vi "Follow Path.vi"(0 "Drivetrain":T10, 1 "Encoder L":T6, 2 "Encoder R":T6, 3 "Gyro":T3 {"Sample Rate" min=0.25 max=100.0 step=0.25}, 4 "Trajectory":T1, 5 "error in":errorcluster, 6 "Queue in":refnum<queue>) -> (19 "error out":errorcluster)   [LabVIEW 2016, in "Drive System.lvlib"]
uses:
  Drive System.lvlib
  DriveCmd.ctl
  DriveCmdList.ctl
  <vilib>/Rock Robotics/WPI/RobotDrive/WPI_RobotDriveDevRef.ctl
  <vilib>/Rock Robotics/WPI/MotorControl/WPI_MotorControlDeviceRef.ctl
  <vilib>/Rock Robotics/WPI/MotorControl/WPI_MotorControlType.ctl
  <vilib>/Rock Robotics/SystemInterfaces/DIO/FPGA_DIOPWMChannel.ctl
  <vilib>/Rock Robotics/WPI/PWM/WPI_PWMDeadband.ctl
  <vilib>/Rock Robotics/WPI/Encoder/WPI_EncoderDevRef.ctl
  <vilib>/Rock Robotics/SystemInterfaces/Encoder/FPGA_EncoderIdx.ctl
  <vilib>/Rock Robotics/SystemInterfaces/Counter/FPGA_CounterCtrSystemIndex.ctl
  <vilib>/Rock Robotics/WPI/Encoder/WPI_EncoderType.ctl
  <vilib>/Rock Robotics/WPI/Gyro/WPI_GyroDevRef.ctl
  <vilib>/Rock Robotics/SystemInterfaces/AI/FPGA_AIChannel.ctl
  <vilib>/Rock Robotics/SystemInterfaces/spilib/spi_bus.ctl
  Varient Cmd Types/Follow Path.ctl
  Pathfinder/VIs/Segment.ctl
  <vilib>/Platform/TimedLoop/XDataNode/timing_clust.ctl
  <vilib>/Platform/TimedLoop/XDataNode/nitl_modes.ctl
  <vilib>/Platform/TimedLoop/XDataNode/wakeup.ctl
  Raw Data.vi
  <vilib>/Platform/TimedLoop/XDataNode/XDataNode.xnode
  <vilib>/Platform/TimedLoop/XDataNode/XDNodeRunTimeDep.lvlib
  Pathfinder/Pathfinder.lvlib
panel:
  in  "Gyro PIDF":cluster{"Kp":dbl, "Ki":dbl, "Kd":dbl, "Kf":dbl} {"Kf" format="%.3f"; "Kd" format="%.3f"; "Ki" format="%.3f"; "Kp" format="%.3f"}
  in  "Gyro iZone":dbl=inf format="%#_13g"
  in  "Gyro Invert":bool
  in  "Gyro output range":cluster{"output high":dbl, "output low":dbl}={"output high"=1.0, "output low"=-1.0} {"output low" format="%.2f"; "output high" format="%.2f"}
  in  "PIDF gains":cluster{"Kp":dbl, "Ki":dbl, "Kd":dbl, "Kf":dbl} {"Kf" format="%.3f"; "Kd" format="%.3f"; "Ki" format="%.3f"; "Kp" format="%.3f"}
  in  "i Zone":dbl=inf format="%.2f"
  in  "invert? (F)":bool
  in  "output range":cluster{"output high":dbl, "output low":dbl}={"output high"=1.0, "output low"=-1.0} {"output low" format="%.2f"; "output high" format="%.2f"}
  in  "Ka":dbl
  in  "Kv":dbl
  # "Analog"
  # "XRS"
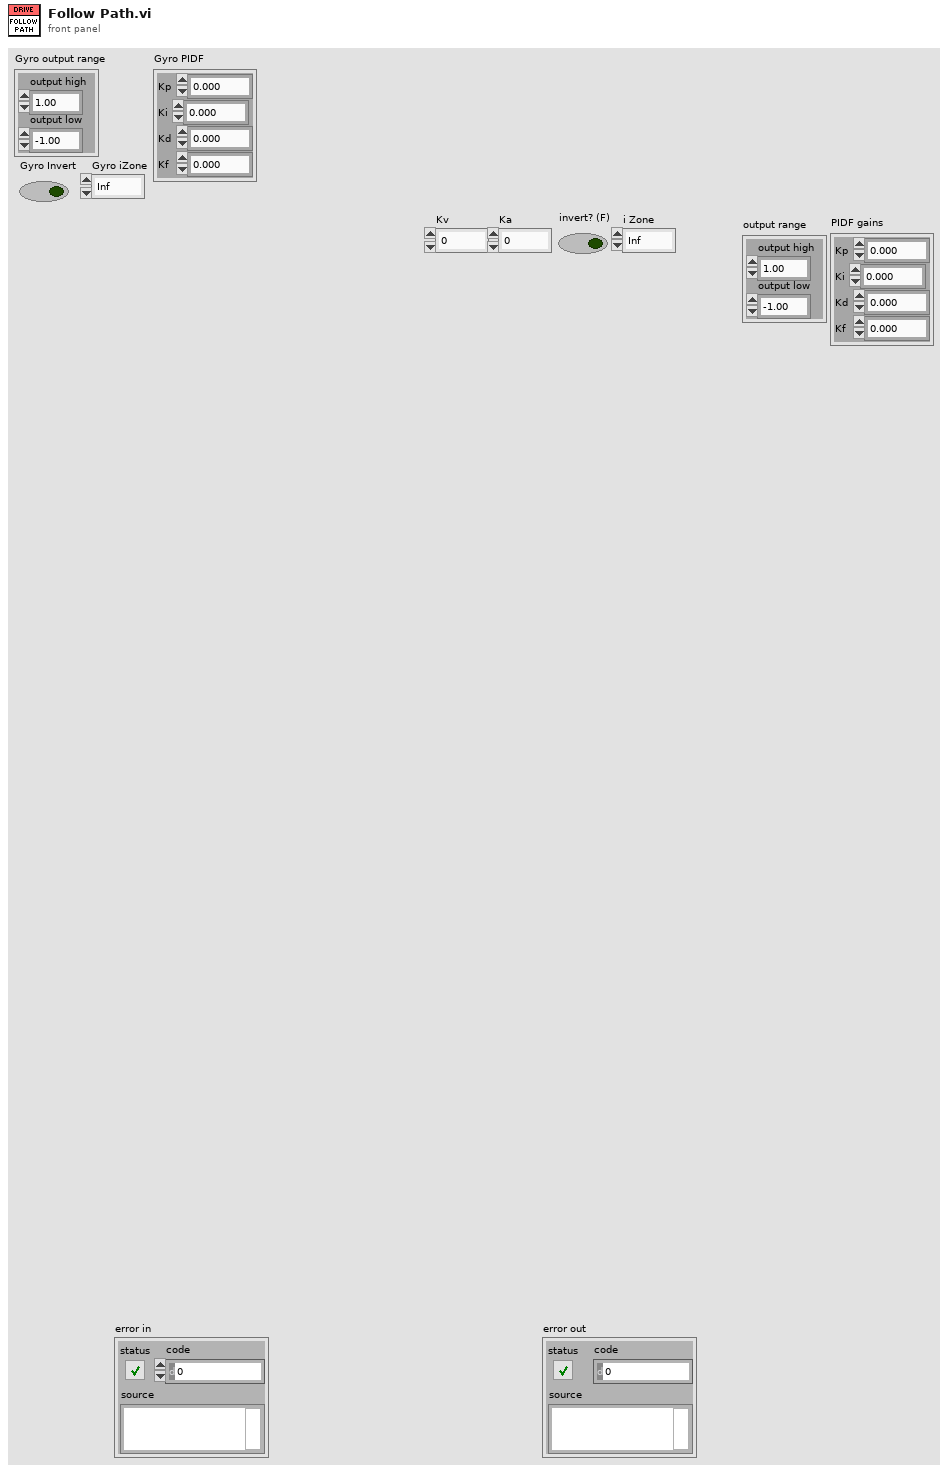
[diagram p1: front panel]
types:
  T1 = typedef "Drive System.lvlib/Follow Path.ctl" = cluster{"Left":T2[], "Right":T2[]}
  T2 = typedef "Pathfinder.lvlib/Segment.ctl" = cluster{"dt":dbl, "x":dbl, "y":dbl, "position":dbl, "velocity":dbl, "acceleration":dbl, "jerk":dbl, "heading":dbl}
  T3 = typedef "WPI_GyroDevRef.ctl" = cluster{"DevStatus":errorcluster, "Analog Channel":T4, "Offset":dbl, "Gain (VoltsPerDegree/Second)":dbl, "Gyro Type":enum16{"Analog", "XRS450"}, "Handle":i32, "SPI Bus":T5, "Device Found":bool, "Sample Rate":dbl, "Calibrate On Open":bool}
  T4 = typedef "FPGA_AIChannel.ctl" = enum8{"AI 0", "AI 1", "AI 2", "AI 3", "AI MXP 0", "AI MXP 1", "AI MXP 2", "AI MXP 3", "Invalid"}
  T5 = typedef "spi_bus.ctl" = enum16{"SPI On-Board, CS0", "SPI On-Board, CS1", "SPI On-Board, CS2", "SPI On-Board, CS3", "SPI MXP", "Invalid"}
  T6 = typedef "WPI_EncoderDevRef.ctl" = cluster{"DevStatus":errorcluster, "EncoderIndex":T7, "CounterIndex":T8, "DistancePerCount":dbl, "Decoding Type":T9}
  T7 = typedef "FPGA_EncoderIdx.ctl" = enum8{"Enc 0", "Enc 1", "Enc 2", "Enc 3", "Enc 4", "Enc 5", "Enc 6", "Enc 7", "Invalid"}
  T8 = typedef "FPGA_CounterCtrSystemIndex.ctl" = enum8{"Ctr 0", "Ctr 1", "Ctr 2", "Ctr 3", "Ctr 4", "Ctr 5", "Ctr 6", "Ctr 7", "Invalid"}
  T9 = typedef "WPI_EncoderType.ctl" = enum16{"1x", "2x", "4x"}
  T10 = typedef "WPI_RobotDriveDevRef.ctl" = cluster{"DevStatus":errorcluster, "Motors[]":T11[], "Square Inputs":bool, "Max Output":dbl}
  T11 = typedef "WPI_MotorControlDeviceRef.ctl" = cluster{"DeviceStatus":errorcluster, "Type":T12, "PWM":cluster{"PWM Channel":T13, "DeadBand":T14}, "CAN":cluster{"Device Number":u8, "SetOutput VI Ref":variant, "GetOutput VI Ref":variant, "Enable VI Ref":variant, "Disable VI Ref":variant, "Data":variant}, "Invert":bool}
  T12 = typedef "WPI_MotorControlType.ctl" = enum16{"PWM", "CAN"}
  T13 = typedef "FPGA_DIOPWMChannel.ctl" = enum8{"PWM 0", "PWM 1", "PWM 2", "PWM 3", "PWM 4", "PWM 5", "PWM 6", "PWM 7", "PWM 8", "PWM 9", "PWM MXP 0", "PWM MXP 1", "PWM MXP 2", "PWM MXP 3", "PWM MXP 4", "PWM MXP 5", "PWM MXP 6", "PWM MXP 7", "PWM MXP 8", "PWM MXP 9", "Invalid"}
  T14 = typedef "WPI_PWMDeadband.ctl" = cluster{"Name":string, "maxPositivePwm":i32, "minPositivePwm":i32, "centerPwm":i32, "maxNegativePwm":i32, "minNegativePwm":i32, "angularRange":u16}
  T15 = cluster{"Queue in":refnum<queue>, "Drivetrain":T10, "Encoder L":T6, "Encoder R":T6, "Gyro":T3}
  T16 = typedef "XDNodeRunTimeDep.lvlib/timing_clust.ctl" = cluster{"Expected End [f-1]":u64, "Actual End [f-1]":u64, "Finished Late? [f-1]":bool, "Expected End [i-1]":u64, "Actual End [i-1]":u64, "Finished Late? [i-1]":bool, "Expected Start [i]":u64, "Actual Start [i]":u64, "Expected Start [f]":u64, "Actual Start [f]":u64, "Source Name":string, "Structure Name":string, "Period":i64, "Deadline":i64, "Offset":i64, "Start":i64, "Priority":i32, "Timeout":i32, "Mode":T17, "Wakeup Reason":T18, "Error":errorcluster, "Source Type":string, "Secondary Source Type":string, "Global End Time":u64, "Global Start Time":u64, "Frame Duration":u64, "Iteration Duration":u64, "Assigned CPU":i32, "I/O Scan Engine Mode":u32}
  T17 = typedef "XDNodeRunTimeDep.lvlib/nitl_modes.ctl" = enum32{"No Change", "Process missed periods, maintain original phase", "Discard missed periods, maintain original phase", "Process missed periods, ignore original phase", "Discard missed periods, ignore original phase"}
  T18 = typedef "XDNodeRunTimeDep.lvlib/wakeup.ctl" = enum32{"Normal", "Aborted", "Asynchronous wakeup", "Timing source error", "Timed loop error", "Timeout"}
  T19 = typedef "Drive System.lvlib/DriveCmd.ctl" = cluster{"cmd":T20, "data":variant, "Force? (F)":bool, "Lock":string}
  T20 = typedef "Drive System.lvlib/DriveCmdList.ctl" = enum16{"Idle", "Cleanup", "Drive For Time", "Follow Path Speed Control", "Follow Path", "Drive Tank", "Drive Arcade", "Unlock", "Lock"}
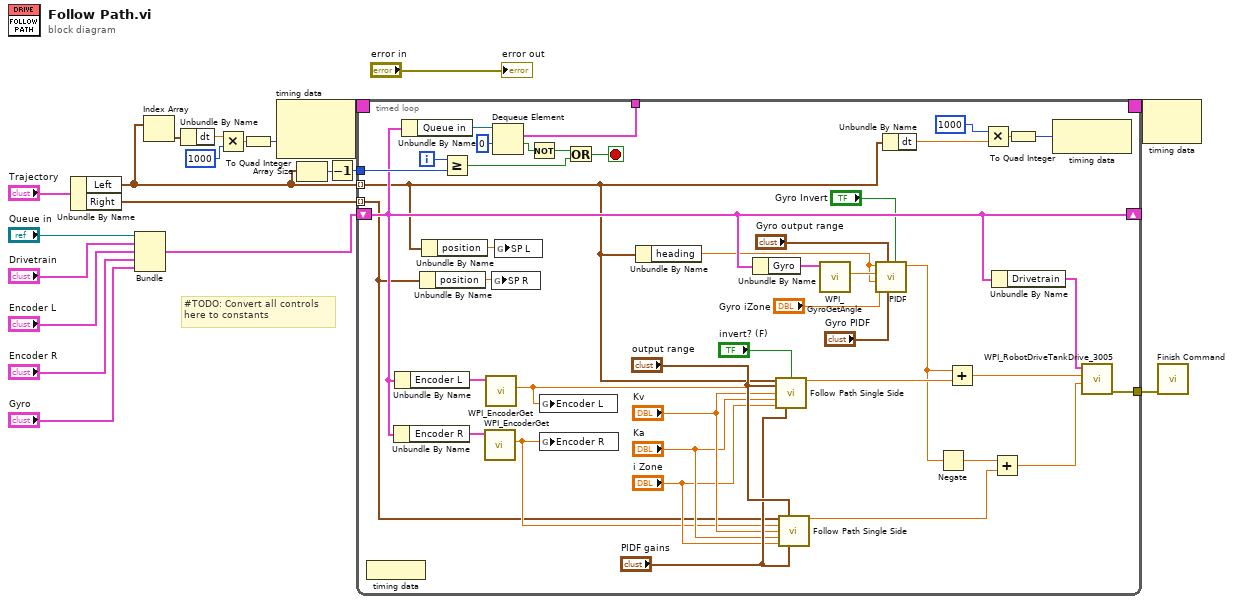
[diagram p0: block diagram]
diagram:
  # "#TODO: Convert all controls\nhere to constants"
  n1 = Unbundle By Name("Trajectory") -> ("Left"=w4:T2[], "Right"=w5:T2[])
  n2 = Bundle("Queue in"="Queue in", "Drivetrain"="Drivetrain", "Encoder L"="Encoder L", "Encoder R"="Encoder R", "Gyro"="Gyro") -> (w7:T15)  [unwired: 1 in]
  n3 = Index Array(array=w4) -> (element=w12:T2)  [unwired: 1 in]
  n4 = Unbundle By Name(w12) -> ("dt"=w11:dbl)
  n5 = Multiply(x=w11, y=i64 1000 ("Period")) -> (x*y=w8:dbl)
  n6 = To Quad Integer(1:w8) -> (0:w9:i64)
  n7 = node-c288(w9) -> (w20:T16)  [unwired: 1 in]
  n8 = Array Size(array=w4) -> (size(s)=w3:i32)
  n9 = Decrement(x=w3) -> (x-1=w2:i32)
  n10 = timed-loop {
    timing: w20 -> [_]
    timing-out: [_] -> w19
    shift-right: [w43] -> _
    shift-left: w7 -> [w43]
    tunnel: w5 -> [w31] mode=indexing
    tunnel: w4 -> [w27] mode=indexing
    tunnel: w2 -> [w56]
    tunnel: [w23] -> w1
    tunnel: [w22] -> _
    i -> [w55]
    stop <- w58 stop-if-true
    n11 = node-c288() -> ()  [unwired: 1 in]
    n12 = Unbundle By Name(w43) -> ("Encoder R"=w48:T6)
    n13 = Unbundle By Name(w43) -> ("Encoder L"=w52:T6)
    n14 = Unbundle By Name(w43) -> ("Queue in"=w61:refnum<queue>)
    n15 = Unbundle By Name(w31) -> ("position"=w30:dbl)
    n16 = Unbundle By Name(w27) -> ("position"=w32:dbl)
    n17 = Greater Or Equal?(x=w55, y=w56) -> (x >= y?=w54:bool)
    n18 = call <vilib>:"WPI_EncoderGet.vi"("EncoderDevRef"=w48) -> ("Distance"=w34:dbl)  [unwired: 5 in, 5 out]
    n19 = call <vilib>:"WPI_EncoderGet.vi"("EncoderDevRef"=w52) -> ("Distance"=w33:dbl)  [unwired: 5 in, 5 out]
    n20 = global write "Raw Data.vi" "SP R"(w30) -> ()
    n21 = Dequeue Element(queue=w61, timeout in ms (-1)=0) -> (element=w22:T19, timed out?=w21:bool)  [unwired: 1 in, 2 out]
    n22 = global write "Raw Data.vi" "SP L"(w32) -> ()
    n23 = Not(x=w21) -> (.not. x?=w57:bool)
    n24 = global write "Raw Data.vi" "Encoder L"(w33) -> ()
    n25 = global write "Raw Data.vi" "Encoder R"(w34) -> ()
    n26 = Or(x=w57, y=w54) -> (x .or. y?=w58:bool)
    n27 = Unbundle By Name(w27) -> ("heading"=w26:dbl)
    n28 = Unbundle By Name(w43) -> ("Gyro"=w42:T3)
    n29 = call "Follow Path Single Side.vi"("segments"=w27, "output range"="output range", "invert? (F)"="invert? (F)", "Encoder"=w33, "Kv"="Kv", "Ka"="Ka", "i Zone"="i Zone", "PIDF gains"="PIDF gains") -> ("output"=w40:dbl)  [unwired: 7 in]
    n30 = call "Follow Path Single Side.vi"("segments"=w31, "output range"="output range", "Encoder"=w34, "Kv"="Kv", "Ka"="Ka", "i Zone"="i Zone", "PIDF gains"="PIDF gains") -> ("output"=w38:dbl)  [unwired: 8 in]
    n31 = call <vilib>:"WPI_GyroGetAngle.vi"("GyroDevRef"=w42) -> ("Angle"=w41:dbl)  [unwired: 6 in, 4 out]
    n32 = call "PIDF.vi"("invert? (F)"="Gyro Invert", "PIDF gains"="Gyro PIDF", "output range"="Gyro output range", "i Zone"="Gyro iZone", "Feedforward"=w26, "process variable"=w41, "setpoint"=w26) -> ("output"=w37:dbl)  [unwired: 2 in, 2 out]
    n33 = Unbundle By Name(w27) -> ("dt"=w53:dbl)
    n34 = Negate(x=w37) -> (-x=w36:dbl)
    n35 = Add(x=w37, y=w40) -> (x+y=w39:dbl)
    n36 = Multiply(x=i64 1000 ("Period"), y=w53) -> (x*y=w63:dbl)
    n37 = Unbundle By Name(w43) -> ("Drivetrain"=w44:T10)
    n38 = Add(x=w36, y=w38) -> (x+y=w35:dbl)
    n39 = To Quad Integer(1:w63) -> (0:w62:i64)
    n40 = node-c288(w62) -> ()  [unwired: 1 out]
    n41 = call "WPI_RobotDriveTankDrive_3005.vi"("Right axis value"=w35, "Left axis value"=w39, "RobotDriveDevRef"=w44) -> ("error out"=w23:errorcluster)  [unwired: 7 in, 1 out]
  }
  n42 = node-c288(w19) -> ()  [unwired: 1 out]
  n43 = call "Finish Command.vi"("error in"=w1) -> ()  [unwired: 10 in, 1 out]
  "error out" <- "error in"
